vi "connect.vi"(8 "error in (no error)":errorcluster, 11 "MQTT1 in":refnum<class "MQTT1.lvclass">) -> (0 "error out":errorcluster, 2 "Message":refnum<user-event>, 3 "MQTT1 out":refnum<class "MQTT1.lvclass">)   [LabVIEW 2015, in "MQTT1.lvclass"]
uses:
  MQTT1.lvclass
  Libraries/mqtt Folder/src/class/mqtt/mqttTypedef/mqttConnectionStatus.ctl
  Libraries/MQTT/MessageTypedef.ctl
  Libraries/mqtt Folder/src/class/mqtt/mqttTXqueue/mqttTXdataQueueFunction.ctl
  Libraries/mqtt Folder/src/class/mqtt/mqttTXqueue/mqttRXsubscriptionEventFunction.ctl
  Libraries/mqtt Folder/src/class/mqtt/mqttTypedef/mqttConnectionFlags.ctl
  Libraries/mqtt Folder/src/class/mqtt/mqttTypedef/mqttWillInformation.ctl
  Libraries/mqtt Folder/src/class/mqtt/mqttTypedef/mqttBroker.ctl
  Libraries/mqtt Folder/src/class/mqtt/mqttTypedef/mqttUserInformation.ctl
  MQTT1.lvclass/MQTT1.ctl
  Libraries/mqtt Folder/src/class/mqtt/mqtt.lvclass
panel:
  out "sessionPresent":bool
  out "connStatus":T1=enum."Connection refused: not authorized"
  out "success":bool
  in  "willQOS":T2(ring)
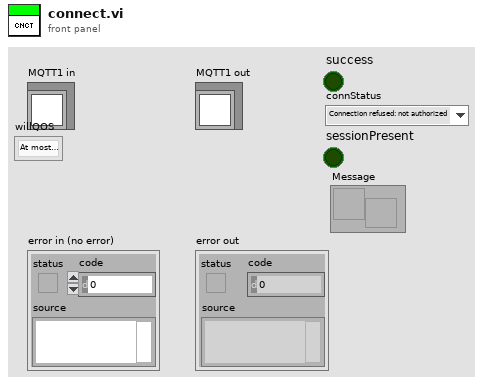
[diagram p1: front panel]
types:
  T1 = typedef "mqttConnectionStatus.ctl" = enum16{"Connection accepted", "Connection refused: unacceptable protocol version", "Connection refused: identifier rejected", "Connection refused: Server unavailable", "Connection refused: bad user name or password", "Connection refused: not authorized"}
  T2 = enum8{"At most once", "At least once", "Exactly once", "Reserved"}
  T3 = typedef "mqttUserInformation.ctl" = cluster{"Will message":string, "Will Topic":string}
  T4 = typedef "mqttBroker.ctl" = cluster{"address":string, "port":u16, "connTimeout":i32, "writeTimeout":i32, "readTimeout":i32, "subTimeout":i32}
  T5 = typedef "mqttWillInformation.ctl" = cluster{"User Name":string, "Password":string}
  T6 = typedef "MessageTypedef.ctl" = cluster{"Topic":string, "Payload":string, "Codename":string}
  T7 = typedef "mqttConnectionFlags.ctl" = cluster{"reserved":bool, "clean session":bool, "will flag":bool, "willQOS":enum8{"At most once", "At least once", "Exactly once", "Reserved"}, "will retain":bool, "password":bool, "user name":bool}
  T8 = typedef "mqttRXsubscriptionEventFunction.ctl" = enum16{"init", "deinit", "getEventRef", "event"}
  T9 = typedef "mqttTXdataQueueFunction.ctl" = enum16{"init", "deinit", "getQueue", "enqueue"}
  T10 = typedef "MQTTclient.lvclass/config.ctl" = cluster{"Broker":cluster{"IP":string, "port":u16, "connTimeout":i32, "writeTimeout":i32, "readTimeout":i32, "subTimeout":i32}, "Connect Flags":cluster{"reserved":bool, "clean session":bool, "will flag":bool, "willQOS":string, "will retain":bool, "password":bool, "user name":bool}, "Keep Alive":u16, "Client Info":cluster{"ClientId":string, "Will Topic":string, "Will Message":string, "User Name":string, "Password":string}}
  T11 = cluster{"IP":string, "port":u16, "connTimeout":i32, "writeTimeout":i32, "readTimeout":i32, "subTimeout":i32}
  T12 = cluster{"reserved":bool, "clean session":bool, "will flag":bool, "willQOS":string, "will retain":bool, "password":bool, "user name":bool}
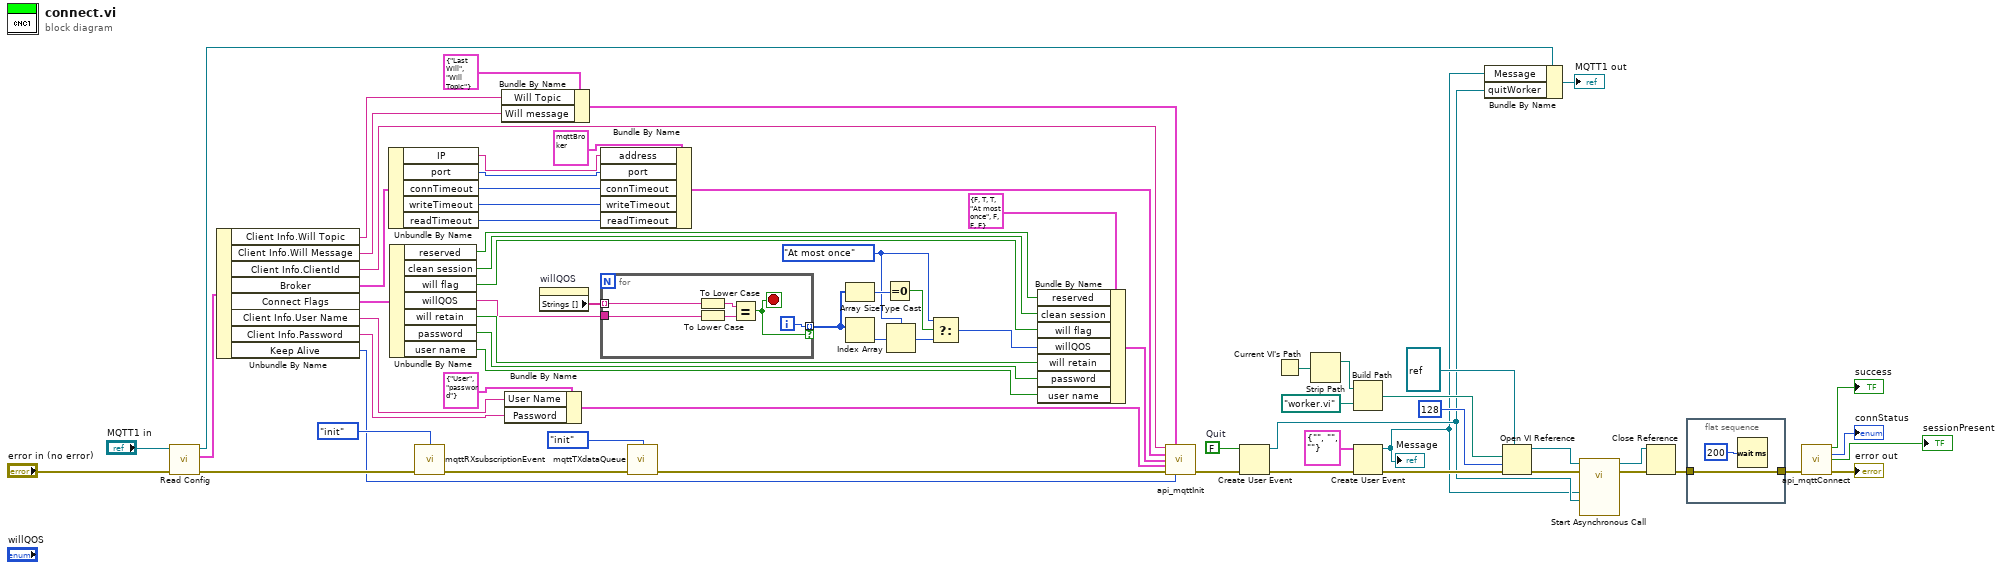
[diagram p0: block diagram]
diagram:
  w41 = FALSE  # Quit
  w44 = T2."At most once" ("willQOS")
  n1 = call-dynamic "Read Config.vi"("error in (no error)"="error in (no error)", "MQTTclient in"="MQTT1 in") -> ("error out"=w64:errorcluster, "Config"=w62:T10, "MQTTclient out"=w28:refnum<class "MQTT1.lvclass">)  [unwired: 7 in]
  n2 = Unbundle By Name(w62) -> ("Client Info.Will Topic"=w1:string, "Client Info.Will Message"=w2:string, "Client Info.ClientId"=w61:string, "Broker"=w13:T11, "Connect Flags"=w60:T12, "Client Info.User Name"=w17:string, "Client Info.Password"=w16:string, "Keep Alive"=w5:u16)
  n3 = Unbundle By Name(w13) -> ("IP"=w12:string, "port"=w11:u16, "connTimeout"=w10:i32, "writeTimeout"=w9:i32, "readTimeout"=w8:i32)
  n4 = Unbundle By Name(w60) -> ("reserved"=w57:bool, "clean session"=w52:bool, "will flag"=w53:bool, "willQOS"=w50:string, "will retain"=w54:bool, "password"=w55:bool, "user name"=w56:bool)
  n5 = call "mqttRXsubscriptionEvent.vi"("function"=mqttRXsubscriptionEventFunction."init", "error in (no error)"=w64) -> ("error out"=w66:errorcluster)  [unwired: 12 in, 1 out]
  n6 = Bundle By Name(cluster=T3 {"Will message"="Last Will", "Will Topic"="Will Topic"} ("Will Info"), "Will Topic"=w1, "Will message"=w2) -> (w3:T3)
  n7 = Bundle By Name(cluster=T5 {"User Name"="User", "Password"="password"} ("User Info"), "User Name"=w17, "Password"=w16) -> (w18:T5)
  n8 = property on="willQOS" class="Enum (strict)"() -> ("Strings []"=w51:string[])  [unwired: 2 in, 2 out]
  n9 = Bundle By Name(cluster=T4 {"address"="localhost", "port"=1883, "connTimeout"=2000, "writeTimeout"=2000, "readTimeout"=2000, "subTimeout"=30000} ("broker"), "address"=w12, "port"=w11, "connTimeout"=w10, "writeTimeout"=w9, "readTimeout"=w8) -> (w14:T4)
  n10 = for {
    tunnel: w51 -> [w75] mode=indexing
    tunnel: w50 -> [w74]
    tunnel: [w71] -> w46 mode=indexing if=w70
    i -> [w71]
    stop <- w70 stop-if-true
    n11 = To Lower Case(string=w75) -> (all lower case string=w73:string)
    n12 = To Lower Case(string=w74) -> (all lower case string=w72:string)
    n13 = Equal?(x=w73, y=w72) -> (x = y?=w70:bool)
  }
  n14 = call "mqttTXdataQueue.vi"("function"=mqttTXdataQueueFunction."init", "error in (no error)"=w66) -> ("error out"=w63:errorcluster)  [unwired: 12 in, 1 out]
  n15 = Array Size(array=w46) -> (size(s)=w49:i32)
  n16 = Index Array(array=w46) -> (element=w45:i32)  [unwired: 1 in]
  n17 = Equal To 0?(x=w49) -> (x = 0?=w48:bool)
  n18 = Type Cast(type=w44, x=w45) -> (*(type *) &x=w43:T2)
  n19 = Select(t=w44, s=w48, f=w43) -> (s? t:f=w47:T2)
  n20 = Bundle By Name(cluster=T7 {"reserved"=FALSE, "clean session"=TRUE, "will flag"=TRUE, "willQOS"=enum."At most once", "will retain"=FALSE, "password"=FALSE, "user name"=FALSE} ("connFlags"), "reserved"=w57, "clean session"=w52, "will flag"=w53, "willQOS"=w47, "will retain"=w54, "password"=w55, "user name"=w56) -> (w58:T7)
  n21 = call "api_mqttInit.vi"("client"=w61, "Will Info"=w3, "broker"=w14, "connFlags"=w58, "User Info"=w18, "error in (no error)"=w63, "keepAlive(sec)"=w5) -> ("error out"=w42:errorcluster)  [unwired: 8 in]
  n22 = Create User Event(user event datatype=w41, error in=w42) -> (user event=w26:refnum<user-event>, error out=w40:errorcluster)
  n23 = Current VI's Path() -> (path=w32:path)
  n24 = Strip Path(path=w32) -> (stripped path=w31:path)  [unwired: 1 out]
  n25 = Build Path(base path=w31, name or relative path=path "worker.vi" ("vi path")) -> (appended path=w29:path)
  n26 = Create User Event(user event datatype=T6 {"Topic"="", "Payload"="", "Codename"=""} ("Message"), error in=w40) -> (user event=w6:refnum<user-event>, error out=w36:errorcluster)
  "Message" <- w6
  n27 = Bundle By Name(cluster=w28, "Message"=w6, "quitWorker"=w26) -> (→"MQTT1 out":refnum<class "MQTT1.lvclass">)
  n28 = Open VI Reference(type specifier VI Refnum (for type only)=refnum<vi> refnum, vi path=w29, options=128, error in (no error)=w36) -> (vi reference=w38:refnum<vi>, error out=w37:errorcluster)  [unwired: 2 in]
  n29 = call-by-ref "Start Asynchronous Call"(reference=w38, error in=w37, "Quit"=w26, "Message"=w6) -> (reference out=w34:refnum<vi>, error out=w33:errorcluster)  [unwired: 9 in, 1 out]
  n30 = Close Reference(reference=w34, error in (no error)=w33) -> (error out=w23:errorcluster)
  n31 = flat-sequence {
    tunnel: [w76] -> w24
    tunnel: w23 -> [w76]
    frame #0 {
      n32 = Wait (ms)(milliseconds to wait=u32 200) -> ()  [unwired: 1 out]
    }
  }
  n33 = call "api_mqttConnect.vi"("error in (no error)"=w24) -> ("success"=→"success":bool, "connStatus"=→"connStatus":T1, "sessionPresent"=→"sessionPresent":bool, "error out"=→"error out":errorcluster)  [unwired: 11 in]
